vi "Turret Auto Align.vi"(9 "Manual Addition":dbl, 10 "AA?":bool) -> (0 "ty":dbl, 1 "tx":dbl, 2 "Turret New Position":dbl)   [LabVIEW 2019]
uses:
  <vilib>/Rock Robotics/Network Tables/NT Read Number.vi
  <vilib>/Rock Robotics/Network Tables/NT Write Number.vi
panel:
  in  "Deadband":dbl=0.1 format="%#_13g"
  in  "Conversion Factor":dbl=0.2
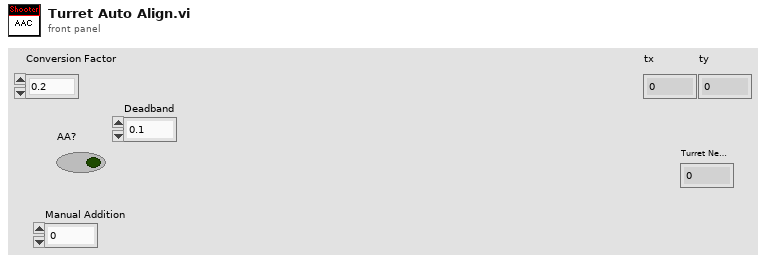
[diagram p1: front panel]
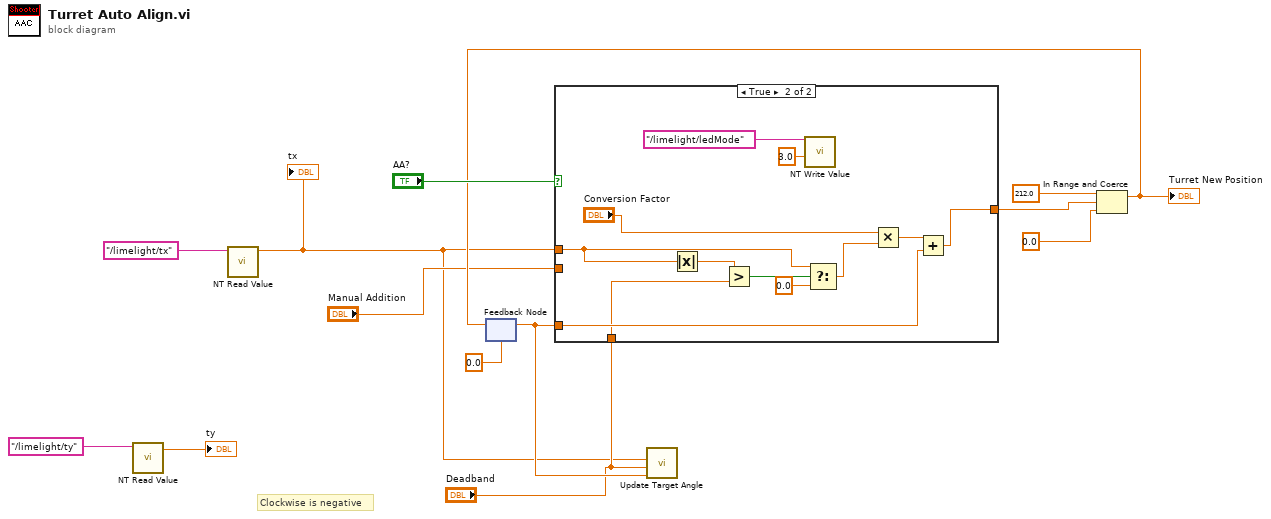
[diagram p0: block diagram]
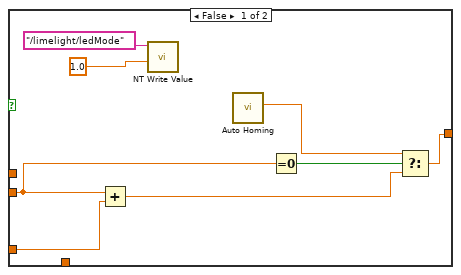
[diagram p2: hidden frame]
diagram:
  # "Clockwise is negative"
  n1 = call-poly <vilib>:"NT Read Value.vi"("Name"="/limelight/ty") -> ("Numeric"=→"ty":dbl)  [unwired: 9 in, 1 out]
  n2 = call-poly <vilib>:"NT Read Value.vi"("Name"="/limelight/tx") -> ("Numeric"=w3:dbl)  [unwired: 9 in, 1 out]
  "tx" <- w3
  n3 = feedback #1(0.0 ("lower limit")) -> (w5:dbl)
  n4 = case shown="True" "AA?" {
    tunnel: w5 -> [w19 w29]
    tunnel: [w16 w28] -> w8
    tunnel: "Manual Addition" -> [w18 _]
    tunnel: "Deadband" -> [_ w23]
    tunnel: w3 -> [_ w22]
    frame False {
      n5 = Add(x=w18, y=w19) -> (x+y=w15:dbl)
      n6 = call-poly <vilib>:"NT Write Value.vi"("Numeric"=1.0, "Name"="/limelight/ledMode") -> ()  [unwired: 9 in, 1 out]
      n7 = call "Auto Homing.vi"() -> ("Turret Angle to go to 2"=w14:dbl)  [unwired: 11 in]
      n8 = Equal To 0?(x=w18) -> (x = 0?=w17:bool)
      n9 = Select(t=w14, s=w17, f=w15) -> (s? t:f=w16:dbl)
    }
    frame True {
      n10 = Absolute Value(x=w22) -> (abs(x)=w27:dbl)
      n11 = Greater?(x=w27, y=w23) -> (0:w26:bool)
      n12 = call-poly <vilib>:"NT Write Value.vi"("Numeric"=3.0, "Name"="/limelight/ledMode") -> ()  [unwired: 9 in, 1 out]
      n13 = Select(t=w22, s=w26, f=0.0) -> (s? t:f=w24:dbl)
      n14 = Multiply(x="Conversion Factor", y=w24) -> (x*y=w30:dbl)
      n15 = Add(x=w30, y=w29) -> (x+y=w28:dbl)
    }
  }
  n16 = call "Update Target Angle.vi"("Turret Position"=w5, "Deadband"="Deadband", "Tx"=w3) -> ()  [unwired: 9 in]
  n17 = In Range and Coerce(upper limit=212.0, x=w8, lower limit=0.0) -> (coerced(x)=w9:dbl)  [unwired: 1 out]
  "Turret New Position" <- w9
  n18 = feedback-in #1(w9) -> ()
